vi "DataSafetyReadGen.vi"(0 "error in":errorcluster) -> (5 "DernColVal":i32, 6 "error out":errorcluster, 7 "LastScanPos":dbl[](array[numeric]), 8 "XY Graph":T1(array[cluster]), 9 "AllYData":dbl[][](array[numeric]))   [LabVIEW 2010]
doc: "Ce VI lit les données contenu dans le fichier de sauvegarde automatique. Ces données correspondent aux valeurs prises lors du dernier balayage. La sauvegarde automatique est effectué après chaque acquisition."
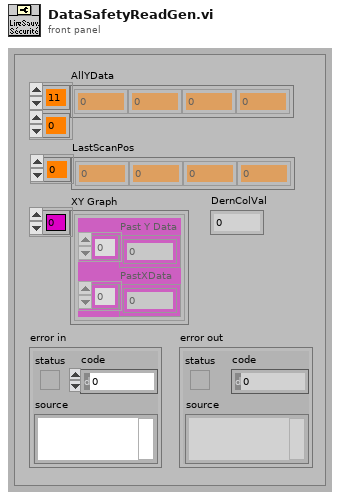
[diagram p1: front panel]
types:
  T1 = cluster{"Past Y Data":dbl[], "PastXData":dbl[]}[]
  T2 = cluster{"AllYData 2":dbl[][], "XY Graph":cluster{"Past Y Data":dbl[], "PastXData":dbl[]}[], "LastScanPos 2":dbl[]}
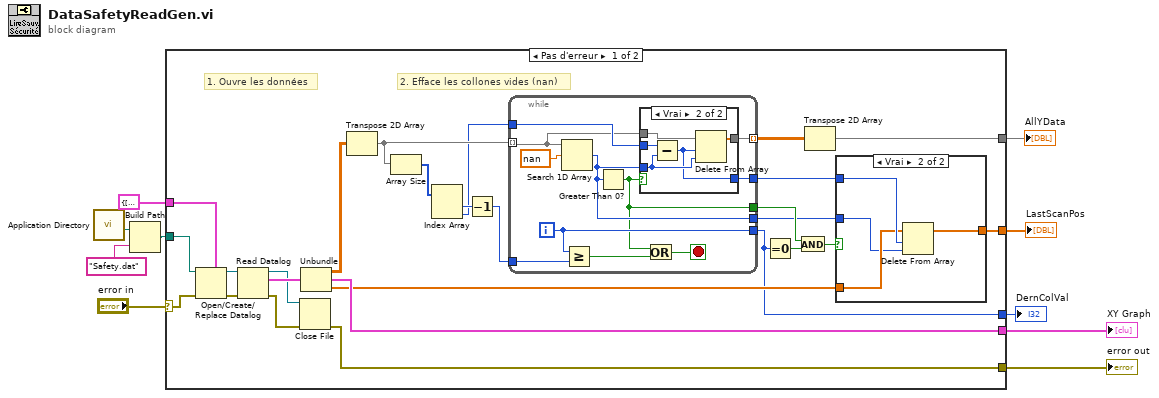
[diagram p0: block diagram]
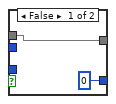
[diagram p3: hidden frame]
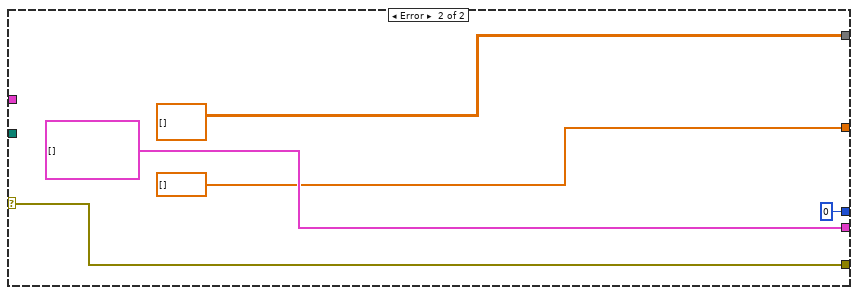
[diagram p4: hidden frame]
diagram:
  n1 = call <vilib>:"Application Directory.vi"() -> ("Application Directory"=w2:path)
  n2 = Build Path(base path=w2, name or relative path="Safety.dat") -> (appended path=w9:path)
  n3 = case shown="Pas d'erreur" "error in" {
    selector: "error in" -> [w29 w61]
    tunnel: w9 -> [w36 _]
    tunnel: T2 {"AllYData 2"=[], "XY Graph"=[], "LastScanPos 2"=[]} ("output cluster") -> [w33 _]
    tunnel: [w28 w61] -> w7
    tunnel: [w17 dbl[][] [] ("AllYData 2")] -> w6
    tunnel: [w31 T1 [] ("XY Graph")] -> w3
    tunnel: [w20 dbl[] [] ("LastScanPos 2")] -> w5
    tunnel: [w12 0] -> w1
    frame No Error {
      # "2. Efface les collones vides (nan)"
      # "1. Ouvre les données"
      n4 = Open/Create/Replace Datalog(5:w33, 8:w29, 11:w36) -> (0:w34:errorcluster, 3:w35:refnum<k1>)  [unwired: 3 in, 1 out]
      n5 = Read Datalog(4:w34, 7:w35) -> (0:w32:errorcluster, 2:w30:T2, 3:w27:refnum<k1>)  [unwired: 1 in]
      n6 = Close File(refnum=w27, error in=w32) -> (error out=w28:errorcluster)  [unwired: 1 out]
      n7 = Unbundle(w30) -> ("AllYData 2"=w21:dbl[][], "XY Graph"=w31:T1, "LastScanPos 2"=w22:dbl[])
      n8 = Transpose 2D Array(2D array=w21) -> (transposed array=w23:dbl[][])
      n9 = Array Size(array=w23) -> (size(s)=w26:i32[])
      n10 = Index Array(array=w26) -> (element #1=w25:i32, element #2=w19:i32)  [unwired: 2 in]
      n11 = Decrement(x=w25) -> (x-1=w24:i32)
      n12 = while {
        tunnel: w23 -> [w48] mode=indexing
        tunnel: [w50] -> w12
        tunnel: w24 -> [w51]
        tunnel: w19 -> [w49]
        tunnel: [w47] -> w18 mode=indexing
        tunnel: [w46] -> w11
        tunnel: [w42] -> w15
        tunnel: [w45] -> w13
        i -> [w50]
        stop <- w44 stop-if-true
        n13 = Search 1D Array(1D array=w48, element=nan ("élément")) -> (index of element=w46:i32)  [unwired: 1 in]
        n14 = Greater Or Equal?(x=w50, y=w51) -> (x >= y?=w43:bool)
        n15 = Greater Than 0?(x=w46) -> (x > 0?=w42:bool)
        n16 = case shown="Vrai" w42 {
          tunnel: w49 -> [_ w59]
          tunnel: w46 -> [_ w57]
          tunnel: w48 -> [w54 w58]
          tunnel: [w54 w56] -> w47
          tunnel: [0 w55] -> w45
          frame False {
          }
          frame True {
            n17 = Subtract(x=w59, y=w57) -> (x-y=w55:i32)
            n18 = Delete From Array(array=w58, length=w55, index=w57) -> (array with subset deleted=w56:dbl[])  [unwired: 1 out]
          }
        }
        n19 = Or(x=w42, y=w43) -> (x .or. y?=w44:bool)
      }
      n20 = Equal To 0?(x=w12) -> (x = 0?=w16:bool)
      n21 = And(x=w15, y=w16) -> (x .and. y?=w14:bool)
      n22 = Transpose 2D Array(2D array=w18) -> (transposed array=w17:dbl[][])
      n23 = case shown="Vrai" w14 {
        tunnel: w22 -> [w37 w40]
        tunnel: [w37 w39] -> w20
        tunnel: w13 -> [_ w41]
        tunnel: w11 -> [_ w38]
        frame False {
        }
        frame True {
          n24 = Delete From Array(array=w40, length=w41, index=w38) -> (array with subset deleted=w39:dbl[])  [unwired: 1 out]
        }
      }
    }
    frame Error {
    }
  }
  "error out" <- w7
  "AllYData" <- w6
  "LastScanPos" <- w5
  "XY Graph" <- w3
  "DernColVal" <- w1
